vi "TestCOMXrootandsquare.vi"() -> ()   [LabVIEW 2012]
panel:
  out "数据":dbl
  in  "数值":dbl format="%#_13g"
  in  "xrootandcubic.IClass1":refnum<k7>
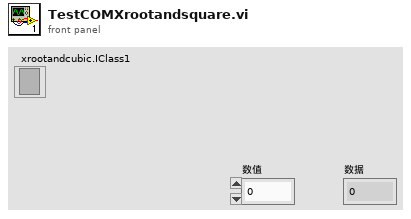
[diagram p1: front panel]
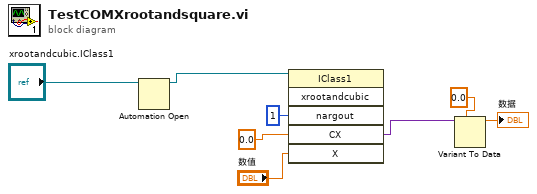
[diagram p0: block diagram]
diagram:
  n1 = Automation Open(Automation Refnum="xrootandcubic.IClass1") -> (Automation Refnum=w7:refnum<k7>)  [unwired: 3 in, 1 out]
  n2 = invoke class="IClass1" method="xrootandcubic"(reference=w7, "nargout"=1, "CX"=0.0, "X"="数值") -> ("CX"=w3:variant)  [unwired: 2 in, 5 out]
  n3 = Variant To Data(type=0.0, Variant=w3) -> (data=→"数据":dbl)  [unwired: 1 in, 1 out]
